vi "insert_into_array.vi"(8 "new element/subarray":u8, 9 "column":u16, 10 "row":u16, 11 "array":u16[](array[numeric])) -> (3 "output array":u16[](array[numeric]))   [LabVIEW 2009]
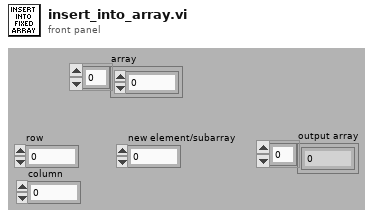
[diagram p1: front panel]
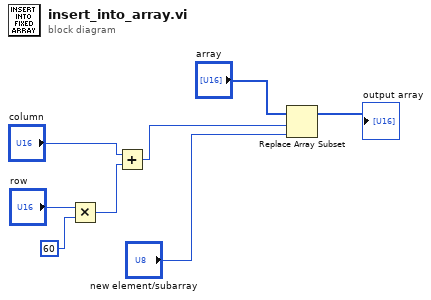
[diagram p0: block diagram]
diagram:
  n1 = Multiply(x="row", y=u16 60) -> (x*y=w5:u16)
  n2 = Add(x="column", y=w5) -> (x+y=w3:u16)
  n3 = Replace Array Subset(array="array", new element="new element/subarray", index=w3) -> (→"output array":u16[])
